vi "批量写入EEPROM.vi"(0 "等待时间（毫秒）":u32, 1 "ID":u32, 2 "CAN通道":u8) -> ()   [LabVIEW 2021]
uses:
  <vilib>/Utility/NIReport.llb/Report Type.ctl
  <vilib>/addons/_office/excel.llb/Excel Get Data ([str]).vi
  <vilib>/Utility/NIReport.llb/NI_report.lvclass
  <vilib>/Utility/NIReport.llb/NI_ReportGenerationCore.lvlib
  <vilib>/addons/_office/NI_ReportGenerationToolkit.lvlib
  <vilib>/Utility/NIReport.llb/Excel/NI_Excel.lvclass
panel:
  out "data":string[][](array[string])
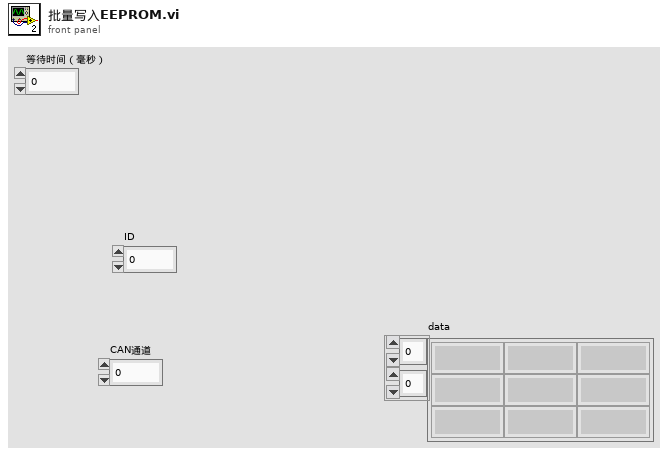
[diagram p1: front panel]
types:
  T1 = typedef "NI_ReportGenerationCore.lvlib/Report Type.ctl" = enum16{"HTML", "Word", "Excel"}
  T2 = cluster{"position (excel)":cluster{"row":i32, "column":i32}, "name (excel)":string, "bookmark (word)":string}
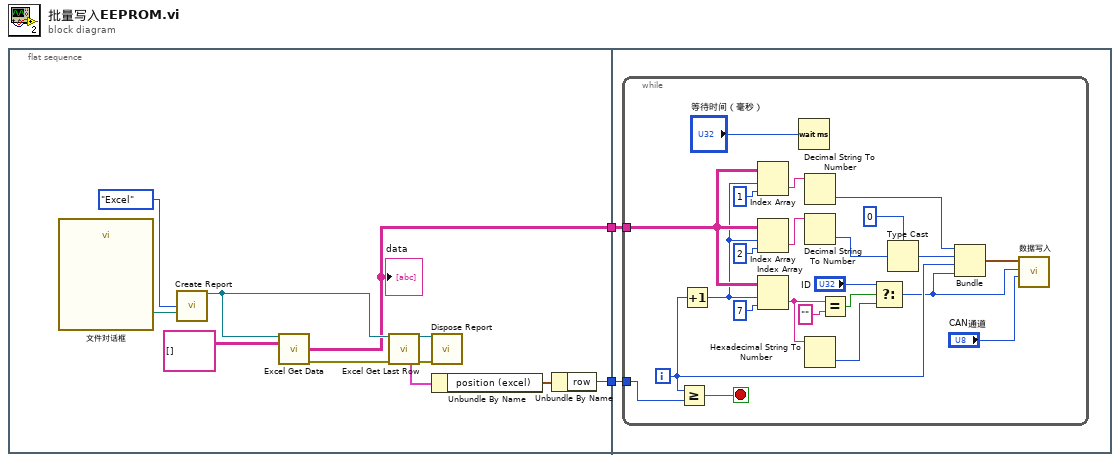
[diagram p0: block diagram]
diagram:
  n1 = flat-sequence {
    tunnel: [w7] -> w2
    tunnel: [w6] -> w1
    tunnel: w2 -> [w15]
    tunnel: w1 -> [w14]
    frame #0 {
      n2 = call "文件对话框"() -> ("selected path"=w12:path)  [unwired: 12 in, 3 out]
      n3 = call <vilib>:"Create Report.vi"("report type"=Report_Type."Excel", "template (empty)"=w12) -> ("report out"=w10:refnum<class "NI_report.lvclass">)  [unwired: 12 in, 1 out]
      n4 = call-poly <vilib>:"Excel Get Data.vi"("report in"=w10, "data type"=string[][] []) -> ("data"=w6:string[][], "error out"=w5:errorcluster)  [unwired: 11 in, 1 out]
      "data" <- w6
      n5 = call <vilib>:"Excel Get Last Row.vi"("report in"=w10, "error in (no error)"=w5) -> ("report out"=w3:refnum<class "NI_report.lvclass">, "MS Office parameters out"=w9:T2, "error out"=w4:errorcluster)  [unwired: 11 in]
      n6 = call-dynamic "Dispose Report.vi"("report in"=w3, "error in (no error)"=w4) -> ()  [unwired: 13 in, 1 out]
      n7 = Unbundle By Name(w9) -> ("position (excel)"=w8:cluster{"row":i32, "column":i32})
      n8 = Unbundle By Name(w8) -> ("row"=w7:i32)
    }
    frame #1 {
      n9 = while {
        tunnel: w15 -> [w31]
        tunnel: w14 -> [w23]
        i -> [w30]
        stop <- w37 stop-if-true
        n10 = Greater Or Equal?(x=w30, y=w31) -> (x >= y?=w37:bool)
        n11 = Increment(x=w30) -> (x+1=w22:i32)
        n12 = Index Array(array=w23, index (row)=w22, index (col)=1 ("禁用的索引 (列)")) -> (element=w35:string)
        n13 = Index Array(array=w23, index (row)=w22, index (col)=2 ("禁用的索引 (列)")) -> (element=w33:string)
        n14 = Index Array(array=w23, index (row)=w22, index (col)=7 ("禁用的索引 (列)")) -> (element=w18:string)
        n15 = Wait (ms)(milliseconds to wait="等待时间（毫秒）") -> ()  [unwired: 1 out]
        n16 = Decimal String To Number(string=w35) -> (number=w32:i32)  [unwired: 2 in, 1 out]
        n17 = Decimal String To Number(string=w33) -> (number=w29:i32)  [unwired: 2 in, 1 out]
        n18 = Hexadecimal String To Number(string=w18) -> (number=w17:u32)  [unwired: 2 in, 1 out]
        n19 = Equal?(x=w18, y="") -> (x = y?=w20:bool)
        n20 = Select(t="ID", s=w20, f=w17) -> (s? t:f=w16:u32)
        n21 = Type Cast(type=u32 0, x=w29) -> (*(type *) &x=w27:u32)
        n22 = Bundle(w32, w27, w30, "ID"=w16) -> (w26:cluster{i32, u32, i32, "ID":u32})  [unwired: 1 in]
        n23 = call "数据写入.vi"("CAN通道"="CAN通道", "ID"=w16, "簇"=w26) -> ()  [unwired: 9 in]
      }
    }
  }
